vi "Chiller Test Konfig.vi"() -> ()   [LabVIEW 2020, in "EPA 1065.lvlib" / "Chiller NO2 1065-376.lvlib"]
uses:
  Chiller NO2 1065-376.lvlib
  Allgemein/allgemeine Sub-VIs.lvlib
  Seiten/FT-IR/FT-IR.lvlib
  Seiten/FT-IR/FGV FT-IR Gasliste Aktionen.ctl
  Messdaten/Aktionen FGV Messdaten.ctl
  Messdaten/Messdaten.lvlib
  Seiten/Grafik/Grafik.lvlib
  EPA 1065.lvlib
  Allgemeine VIs/Aktion Wertaenderung Gasliste.ctl
  Allgemeine VIs/Aktion Test Status.ctl
  Sprachverwaltung/Sprachverwaltung.lvlib
  Sprachverwaltung/FGV Aktion Tabelle zerlegen.ctl
  Aktion FGV Chiller Test.ctl
  Allgemeine VIs/Aktion Registerkarten ein-ausblenden.ctl
  Funktionstasten/Funktionstasten.lvlib
  Funktionstasten/Funktionstasten-Aktion.ctl
  Funktionstasten/Zustaende.ctl
  T90 1065-308/Ergebnis.ctl
  T90 1065-308/T90 Test 1065-308.lvlib
  PDF_Interface/PDF Interface Helper/PDFResultPictures.ctl
  PDF_Interface/PDF Interface Helper/PDF Interface Helper.lvlib
  Visualisierungs Elemente/Zahlen-Ausgabefeld.ctl
  Visualisierungs Elemente/Auswahlfeld.ctl
  Chiller Konfig Daten.ctl
  Messdaten.ctl
panel:
  out "Ergebnis PDF FALSE":T1 caption="Ergebnis 2"
  out "Ergebnis PDF TRUE":T1 caption="Ergebnis 1"
  out "Daten":T2
  out "Messdaten":sgl[](array[numeric])
  in  "Gasliste geändert":bool
  in  "Registerkarte":T3(tab)
  in  "Abbrechen":bool caption="Cancel"
  in  "Test Start":bool
  in  "Chiller Konfig Daten":T4={"Bearbeiter:"="", "Gasflaschen Nr.:"="", "Accuracy"=0.0, "Sollwert"=0.0, "Messgerät:"="", "Seriennummer:"="", "Pfad:"=path "D:/IAG_Data/Log", "Textname:"="", "Einheit"="", "Expiry Date"=timestamp(0 s since 1904-01-01), "Water Concentration:"=0.0, "Componente:"=""} caption="T90 Konfig Daten" {"Expiry Date" format="%<%x>T"}
  in  "Speichern":bool caption="Save"
  out "NOx":T5=1 caption="Gas 4"
  out "Mwert NOx":sgl caption="Mwert" format="%.3f"
  out "PMwert NOx":sgl caption="PMwert" format="%.3f"
  out "NOx":T6 caption="Konzentration" format="%#.3f"
  out "Graph NOx":waveform(dbl)(graph) caption="Graph1"
  out "NO2":T5=1 caption="Gas 4"
  out "Mwert NO2":sgl caption="Mwert" format="%.3f"
  out "PMwert NO2":sgl caption="PMwert" format="%.3f"
  out "NO2":T6 caption="Konzentration" format="%#.3f"
  out "Graph NO2":waveform(dbl)(graph) caption="Graph1"
  in  "xNOxRef aufzeichnen":bool caption="Test Start"
  out "Countdown Anzeige 2":dbl format="%<%M:%S>T"
  in  "H2O aufgeschalten":bool caption="Test Start"
  out "Timeline":u8(slide) scale=0.0..30.0
  out "Countdown Anzeige":dbl format="%<%M:%S>T"
  out "H2O":T5=1 caption="Gas 4"
  out "Mwert H2O":sgl caption="Mwert" format="%.3f"
  out "PMwert H2O":sgl caption="PMwert" format="%.3f"
  out "H2O 2":T6 caption="Konzentration" format="%#.3f"
  out "Graph H2O":waveform(dbl)(graph) caption="Graph1"
  out "NOx 2":T5=1 caption="Gas 4"
  out "Mwert NOx 2":sgl caption="Mwert" format="%.3f"
  out "PMwert NOx 2":sgl caption="PMwert" format="%.3f"
  out "NOx 2":T6 caption="Konzentration" format="%#.3f"
  out "Graph NOx 2":waveform(dbl)(graph) caption="Graph1"
  out "Mwert H2O 2":sgl caption="Mwert" format="%.3f"
  out "PMwert H2O 2":sgl caption="PMwert" format="%.3f"
  out "H2O 2":T6 caption="Konzentration" format="%#.3f"
  out "Graph H2O 2":waveform(dbl)(graph) caption="Graph1"
  in  "xNOxmeas aufzeichnen":bool caption="Test Start"
  out "Countdown Anzeige 3":dbl format="%<%M:%S>T"
  out "H2O":string caption="%"
  out "xNOxmeas":string caption="ppm"
  out "Ergebnis 1":T1
  out "xNOxmeas_dry":string caption="ppm"
  out "xNOxRef":string caption="ppm"
  out "Ergebnis:":string caption="Result:"
  in  "Print PDF":bool caption="Cancel"
  # "Chiller Test EPA CRF40 §1065.376"
  # "General Settings"
  # "Protocol Settings"
  # "%"
  # "%"
  # "NOx"
  # "±"
  # "x"
  # "NO2"
  # "±"
  # "x"
  # "Saturate the gas cooler with H2O by applying vapor to the measuring input and push the button \"H2O connected\""
  # "H2O"
  # "±"
  # "x"
  # "NOx"
  # "±"
  # "x"
  # "H2O"
  # "±"
  # "x"
  # "xNOxmeas_dry ="
  # "/"
  # "(1-"
  # "/ 100)"
  # "x 0.95"
  # "<"
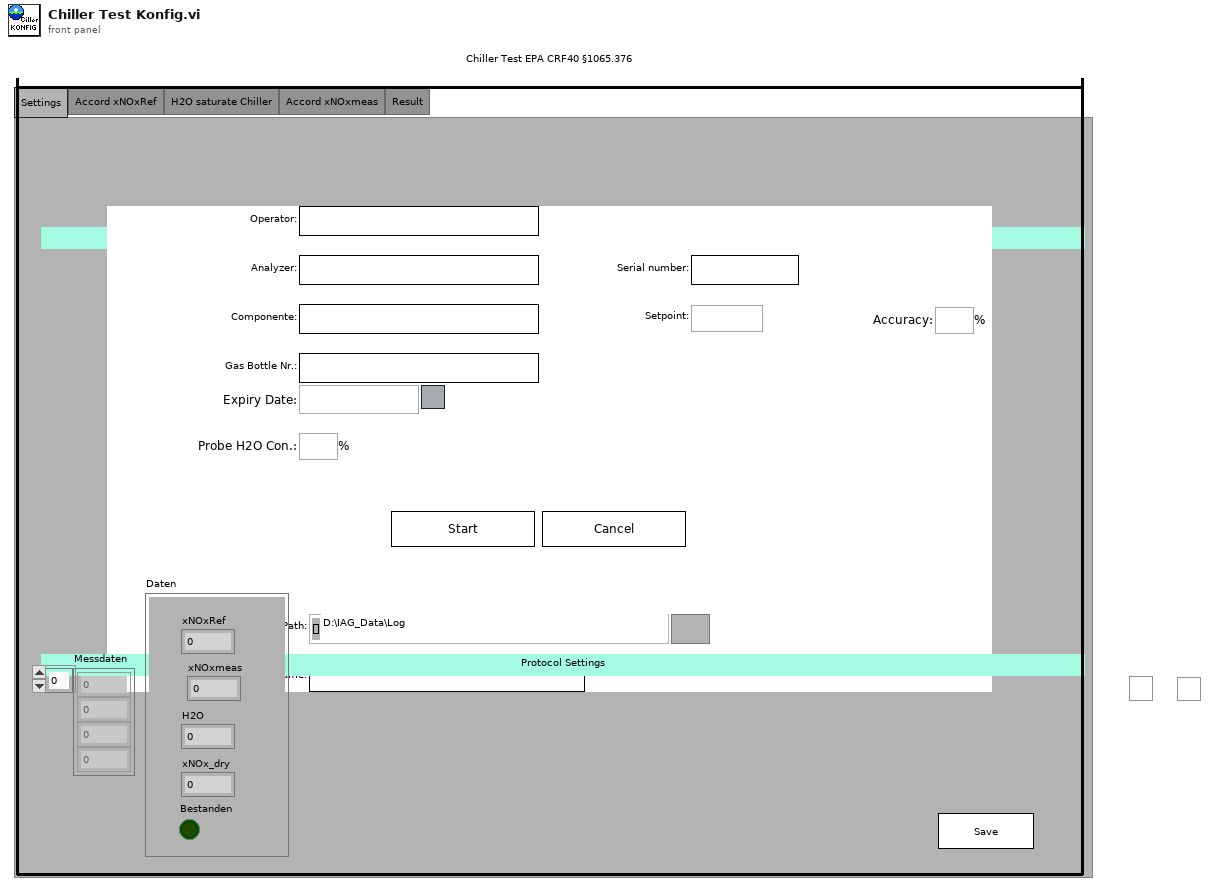
[diagram p1: front panel]
types:
  T1 = typedef "EPA 1065.lvlib/T90 Test 1065-308.lvlib/Ergebnis.ctl" = bool
  T2 = typedef "EPA 1065.lvlib/Chiller NO2 1065-376.lvlib/Messdaten.ctl" = cluster{"xNOxRef":dbl, "xNOxmeas":dbl, "H2O":dbl, "xNOx_dry":dbl, "Bestanden":bool}
  T3 = enum32{"Settings", "Accord xNOxRef", "H2O saturate Chiller", "Accord xNOxmeas", "Result"}
  T4 = typedef "EPA 1065.lvlib/Chiller NO2 1065-376.lvlib/Chiller Konfig Daten.ctl" = cluster{"Bearbeiter:":string, "Gasflaschen Nr.:":string, "Accuracy":dbl, "Sollwert":dbl, "Messgerät:":string, "Seriennummer:":string, "Pfad:":path, "Textname:":string, "Einheit":string, "Expiry Date":timestamp, "Water Concentration:":dbl, "Componente:":string}
  T5 = typedef "Auswahlfeld.ctl" = u16
  T6 = typedef "Zahlen-Ausgabefeld.ctl" = sgl
  T7 = typedef "EPA 1065.lvlib/Chiller NO2 1065-376.lvlib/Aktion FGV Chiller Test.ctl" = enum16{"lesen", "Konfig Daten", "Messdaten", "Resultat", "Daten löschen", "PDF einstellen", "laden", "speichern"}
  T8 = typedef "FT-IR.lvlib/FGV FT-IR Gasliste Aktionen.ctl" = enum16{"lesen", "Gasliste FT-IR", "Gasliste ausgelesen", "laden", "speichern", "löschen"}
  T9 = typedef "EPA 1065.lvlib/Aktion Registerkarten ein-ausblenden.ctl" = enum16{"init", "alle ausblenden", "Seite einblenden", "alle einblenden", "Seite deaktivieren", "Seiten aktivieren"}
  T10 = typedef "Sprachverwaltung.lvlib/FGV Aktion Tabelle zerlegen.ctl" = enum16{"laden", "vereinzeln", "speichern"}
  T11 = typedef "PDF Interface.lvlib/PDF Interface Helper.lvlib/PDFResultPictures.ctl" = cluster{"Yes Ctl Refnum":refnum<vi>, "No Ctl Refnum":refnum<vi>}
  T12 = typedef "String - Ausgabefeld.ctl" = string
  T13 = typedef "EPA 1065.lvlib/Aktion Test Status.ctl" = enum16{"init", "lesen", "prüfen", "Interference 366", "Interference 375", "Chiller läuft", "Drift läuft", "Pre Test läuft", "FID Optimization läuft", "FID Interference läuft", "HovaCAL Interference", "LinV2"}
  T14 = typedef "EPA 1065.lvlib/Aktion Wertaenderung Gasliste.ctl" = enum16{"Init", "lesen", "Gasliste geändert", "ARN inaktiv", "LEAK inaktiv", "Interference 366 inaktiv", "T90 inaktiv", "Interference 375 inaktiv", "Chiller inaktiv", "FID O2 inaktiv", "FID Opti inaktiv", "Drift inaktiv", "Pre Test inaktiv", "LinV2 inaktiv", "HovaCAL Interference inaktiv"}
  T15 = typedef "Messdaten.lvlib/Aktionen FGV Messdaten.ctl" = enum16{"lesen", "schreiben", "löschen", "Mittelwerte", "Komponente"}
  T16 = typedef "Funktionstasten.lvlib/Zustaende.ctl" = enum16{"Standby", "Pause", "Eco", "Messen", "Kalibrieren", "Spülen Filter", "Spülen Leitung", "Umgebungsluft", "0-Gas", "Cal-Gas", "CG zu PNS", "-------------", "Init 1", "Init 2", "Init 3", "Init 4", "Messen vorbereiten", "Messen durchführen", "Exit"}
  T17 = typedef "Funktionstasten.lvlib/Funktionstasten-Aktion.ctl" = enum16{"Initialisieren", "Zustand setzen", "Taste gedrückt", "Fehler speichern", "Lesen", "Manuell", "Remote", "Bitparallel", "Samplepoint", "Zeit Prüfen", "reset Umschalten"}
  T18 = typedef "EPA 1065.lvlib/Aktive Tests Cluster.ctl" = cluster{"ANR läuft":bool, "T90 läuft":bool, "Leak läuft":bool, "Interference 366 läuft":bool, "Interference 375 läuft":bool, "Chiller läuft":bool, "FID Interference läuft":bool, "FID optimization läuft":bool, "Drift läuft":bool, "Pre-test läuft":bool, "HovaCAL Interference läuft":bool, "LinV2 läuft":bool}
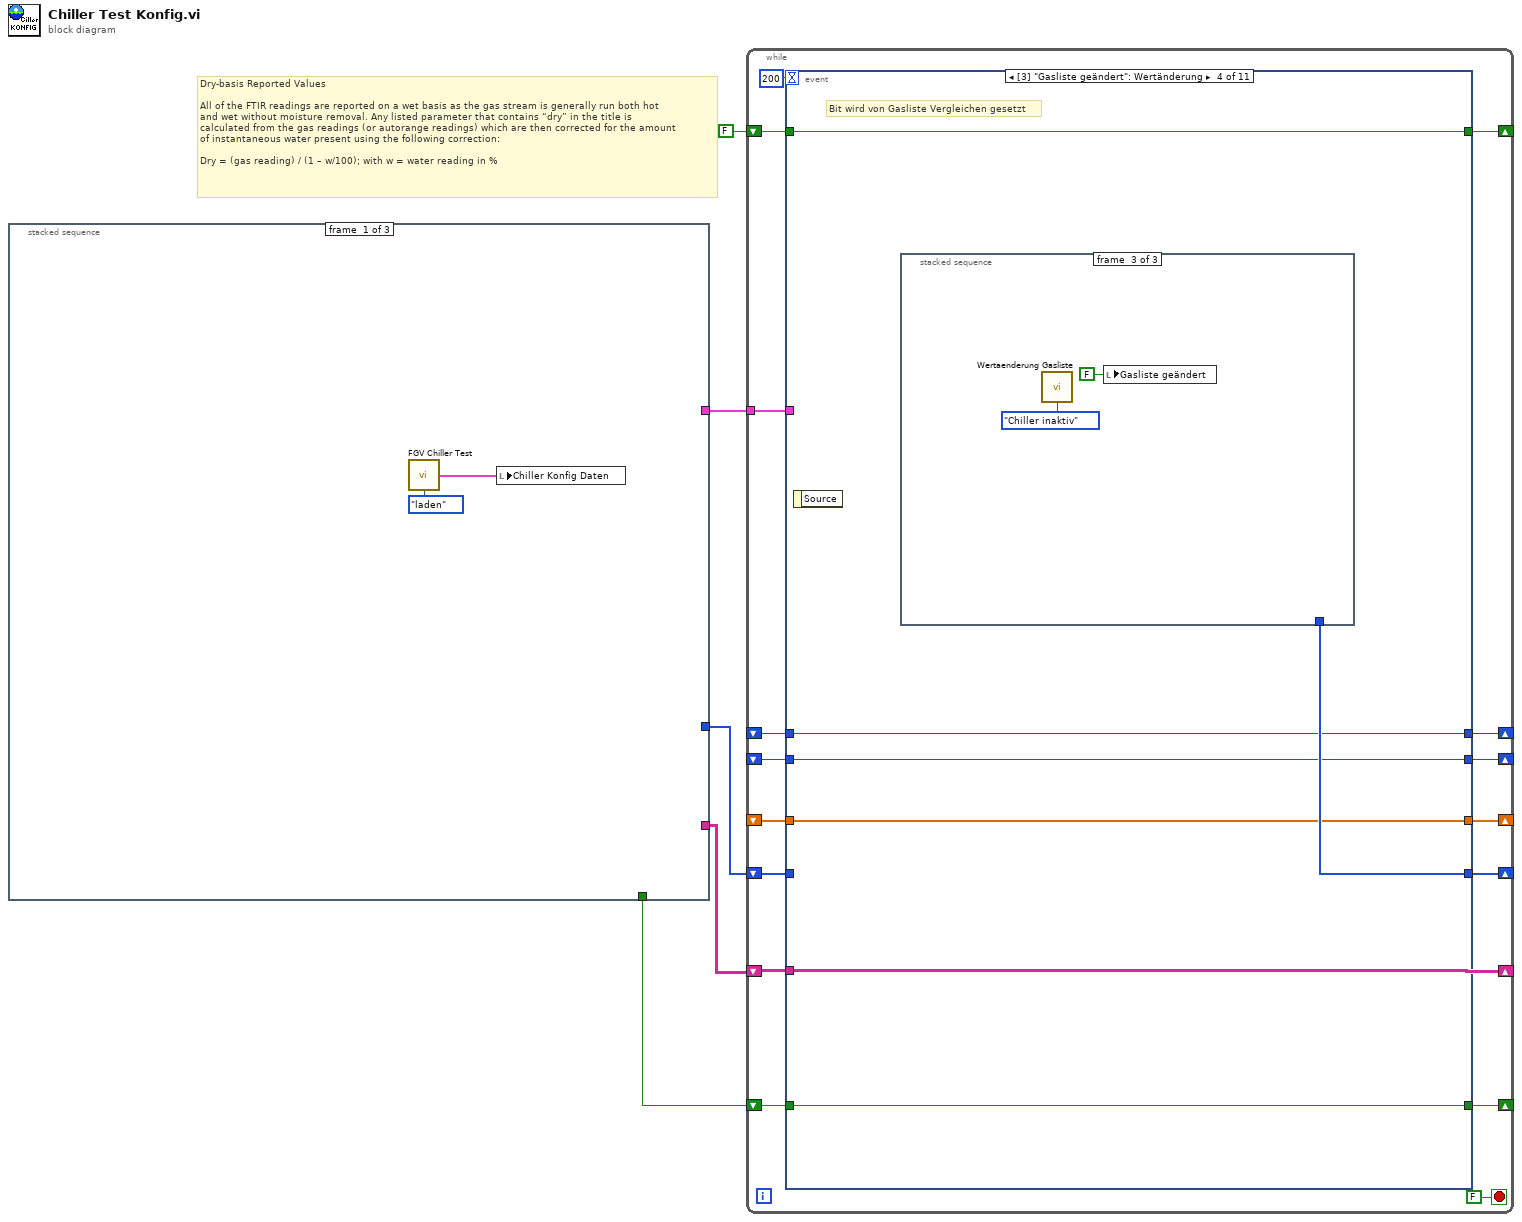
[diagram p0: block diagram]
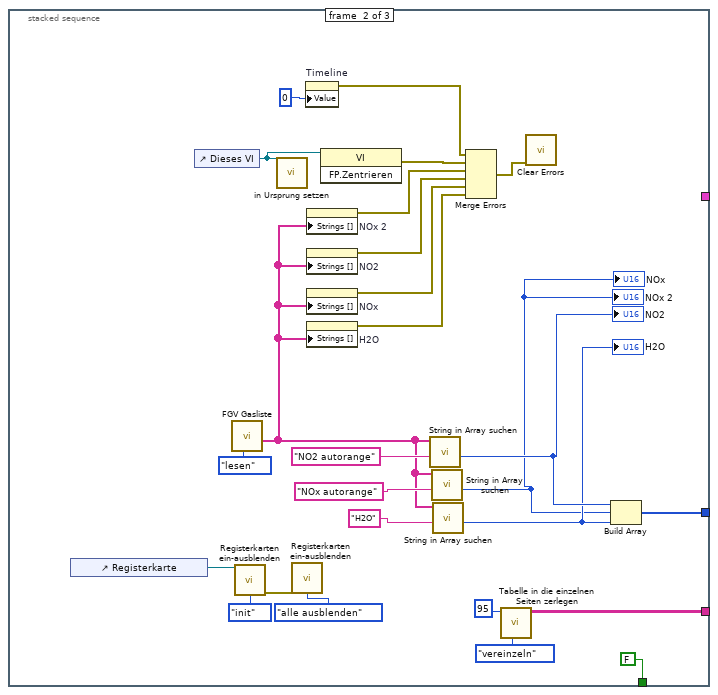
[diagram p2: hidden frame]
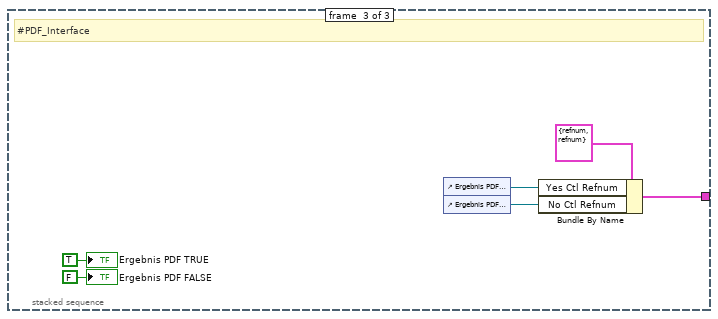
[diagram p3: hidden frame]
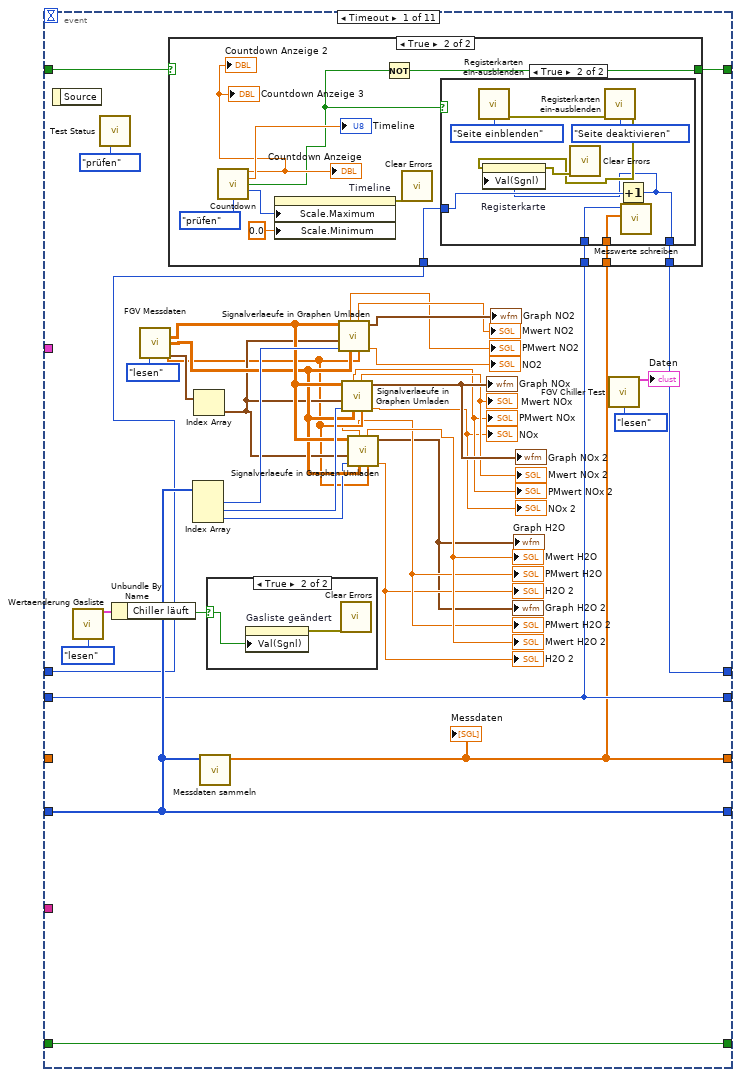
[diagram p4: hidden frame]
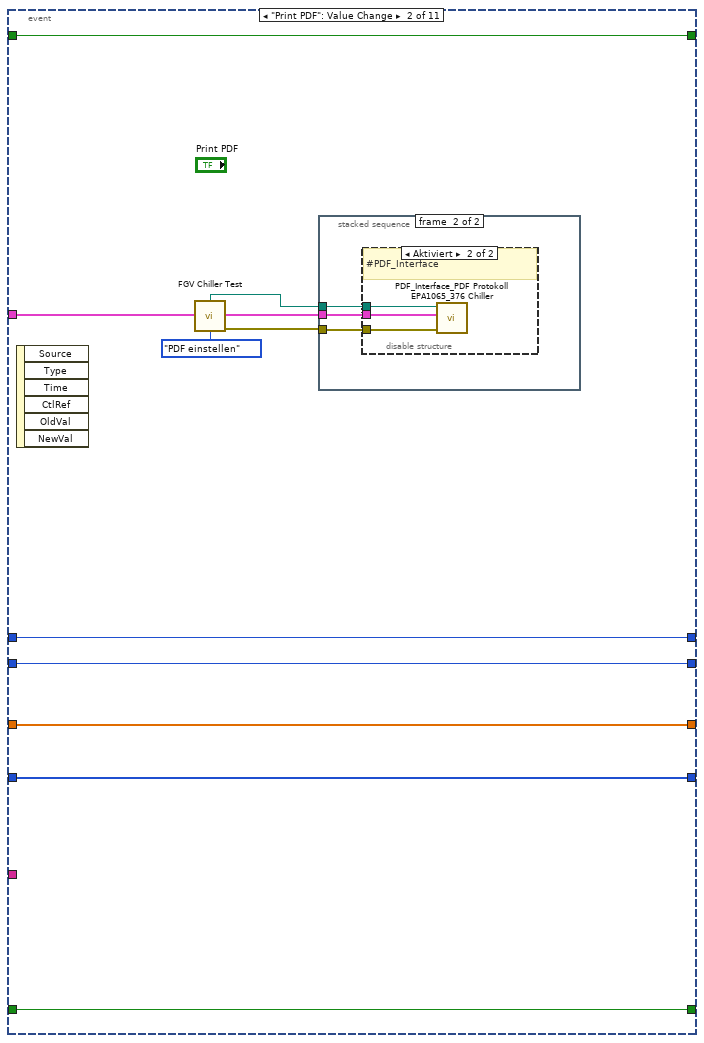
[diagram p8: hidden frame]
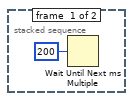
[diagram p9: hidden frame]
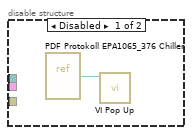
[diagram p10: hidden frame]
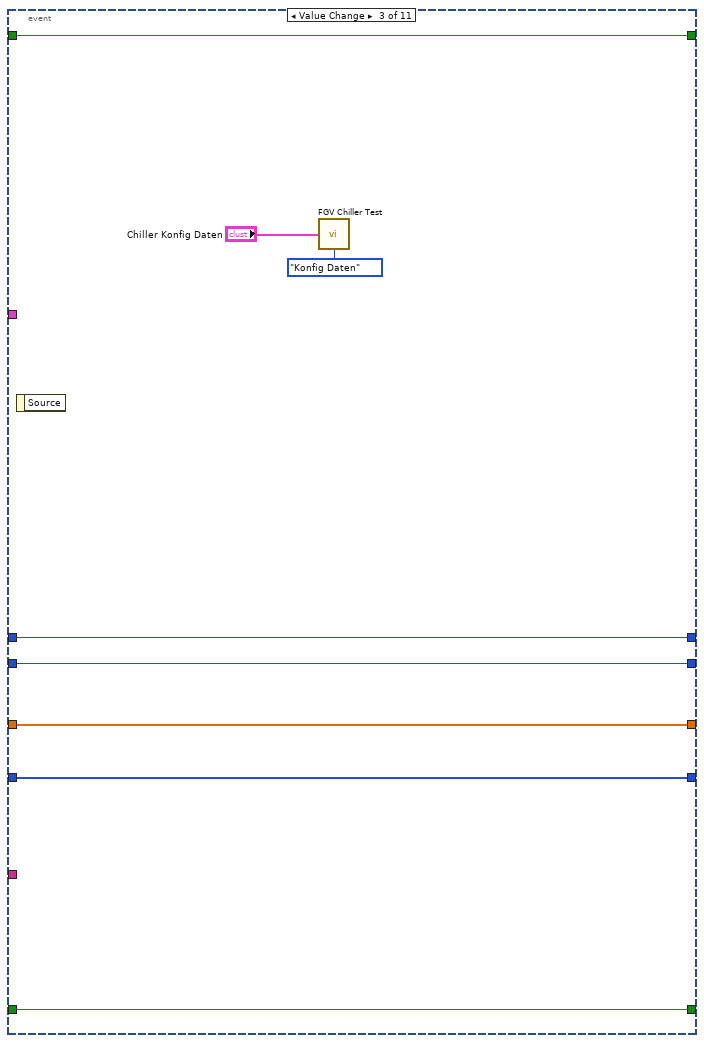
[diagram p11: hidden frame]
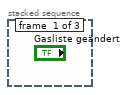
[diagram p12: hidden frame]
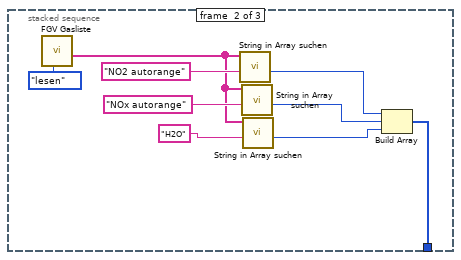
[diagram p13: hidden frame]
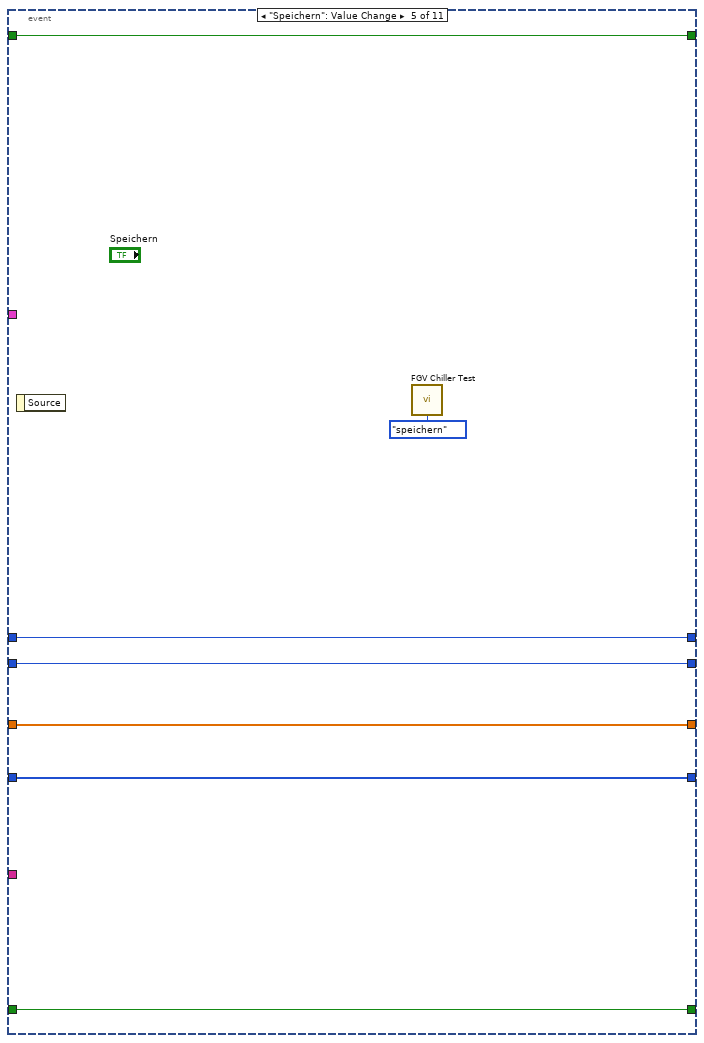
[diagram p14: hidden frame]
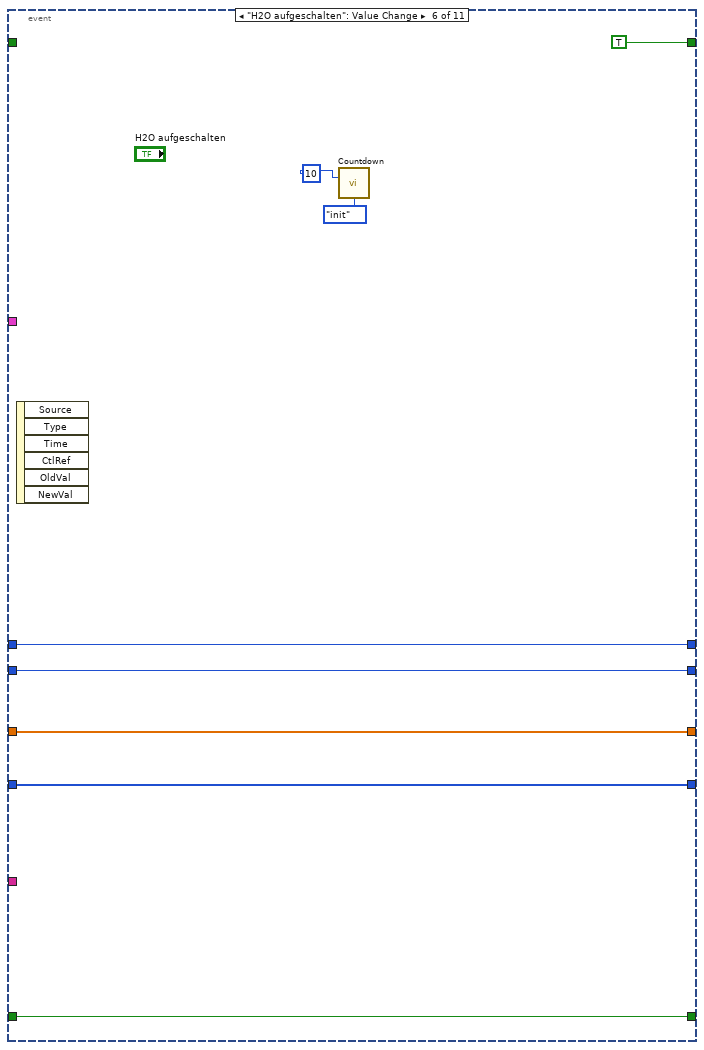
[diagram p15: hidden frame]
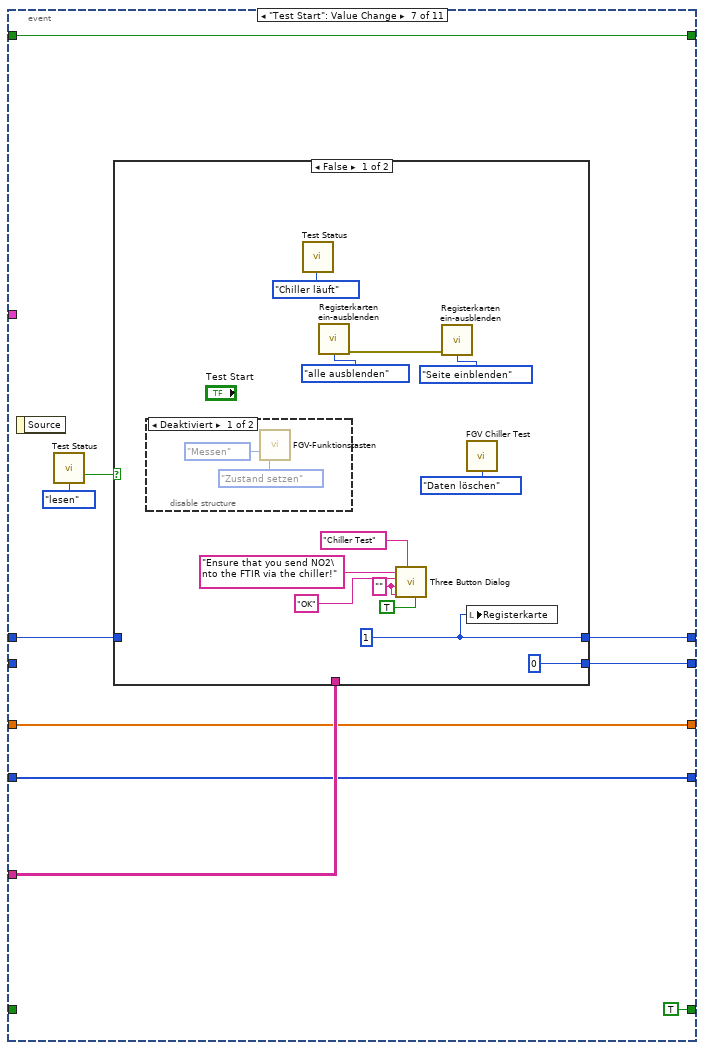
[diagram p16: hidden frame]
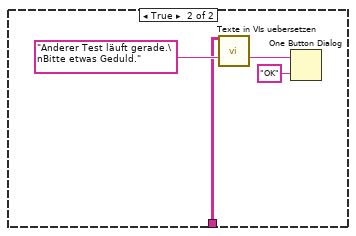
[diagram p18: hidden frame]
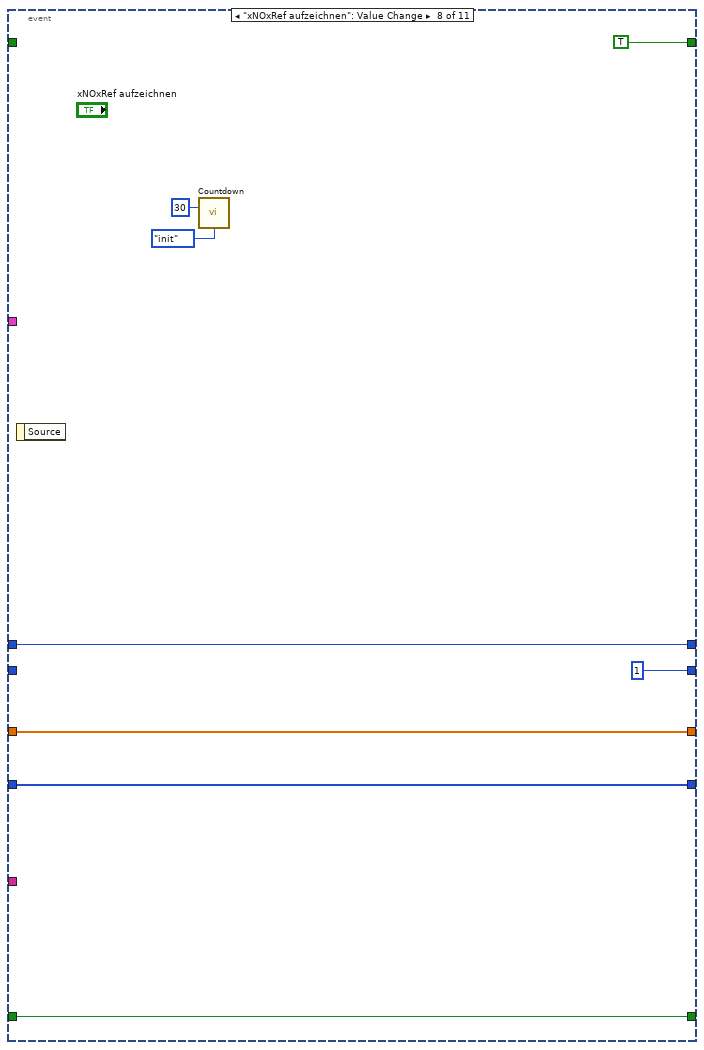
[diagram p19: hidden frame]
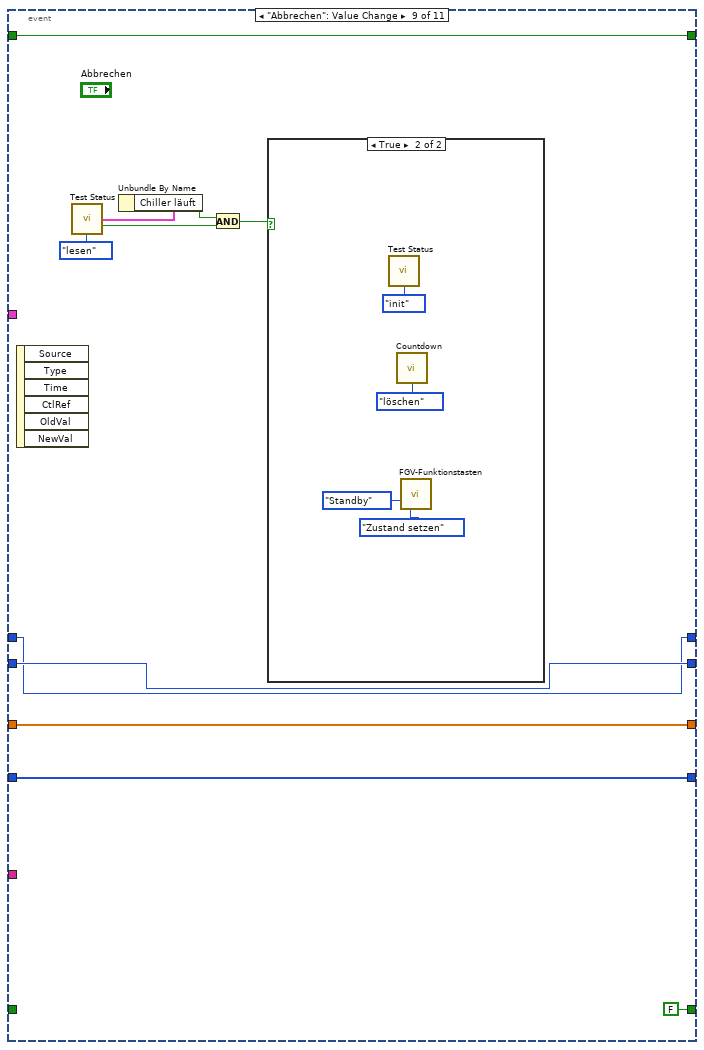
[diagram p20: hidden frame]
diagram:
  # "Dry-basis Reported Values\n\nAll of the FTIR readings are reported on a wet basis as the gas stream is generally run both hot\nand wet without moisture removal. Any listed parameter that contains “dry” in the title is\ncalculated from the gas readings (or autorange readings) which are then corrected for the amount\nof instantaneous water present using the following correction:\n\nDry = (gas reading) / (1 – w/100); with w = water reading in %"
  n1 = stacked-sequence {
    tunnel: [_ w28 _] -> w5
    tunnel: [_ w17 _] -> w3
    tunnel: [_ FALSE _] -> w2
    tunnel: [_ _ w34] -> w1
    frame #0 {
      n2 = call "FGV Chiller Test.vi"("Aktion"=Aktion_FGV_Chiller_Test."laden") -> ("Chiller Konfig Daten"=w6:T4)  [unwired: 11 in, 3 out]
      n3 = local write "Chiller Konfig Daten"(w6) -> ()
    }
    frame #1 {
      n4 = control-ref of="Registerkarte"() -> (w24:refnum<vi>)
      n5 = control-ref of="Dieses VI"() -> (w32:refnum<vi>)
      n6 = call "FGV Gasliste.vi"("Aktionen"=FGV_FT-IR_Gasliste_Aktionen."lesen") -> ("Aktuelle Gasliste gesamt"=w16:T12[])  [unwired: 8 in, 2 out]
      n7 = call "Registerkarten ein-ausblenden.vi"("Registerkartenreferenz"=w24, "Aktion"=Aktion_Registerkarten_ein-ausblenden."init") -> ("error out"=w22:errorcluster)  [unwired: 13 in]
      n8 = call "in Ursprung setzen.vi"("VI Referenz"=w32) -> ()  [unwired: 10 in, 1 out]
      n9 = call "Registerkarten ein-ausblenden.vi"("error in (no error)"=w22, "Aktion"=Aktion_Registerkarten_ein-ausblenden."alle ausblenden") -> ()  [unwired: 13 in, 1 out]
      n10 = property on="Timeline" class="Schieber (strikt)"("Value"=u8 0 ("Timeline")) -> (error out=w26:errorcluster)  [unwired: 2 in, 1 out]
      n11 = property on="NOx 2" class="Ring (strikt)"("Strings []"=w16) -> (error out=w15:errorcluster)  [unwired: 2 in, 1 out]
      n12 = property on="NO2" class="Ring (strikt)"("Strings []"=w16) -> (error out=w14:errorcluster)  [unwired: 2 in, 1 out]
      n13 = property on="NOx" class="Ring (strikt)"("Strings []"=w16) -> (error out=w13:errorcluster)  [unwired: 2 in, 1 out]
      n14 = property on="H2O" class="Ring (strikt)"("Strings []"=w16) -> (error out=w12:errorcluster)  [unwired: 2 in, 1 out]
      n15 = invoke class="VI" method="FP.Zentrieren"(reference=w32) -> (error out=w31:errorcluster)  [unwired: 2 in, 2 out]
      n16 = call "String in Array suchen.vi"("Nach String/Zeichen suchen (-)"="NO2 autorange", "String-Array"=w16) -> ("Index"=w11:i32)  [unwired: 7 in, 2 out]
      "NO2" <- w11
      n17 = call "String in Array suchen.vi"("Nach String/Zeichen suchen (-)"="NOx autorange", "String-Array"=w16) -> ("Index"=w8:i32)  [unwired: 7 in, 2 out]
      "NOx 2" <- w8
      "NOx" <- w8
      n18 = call "String in Array suchen.vi"("Nach String/Zeichen suchen (-)"="H2O", "String-Array"=w16) -> ("Index"=w10:i32)  [unwired: 7 in, 2 out]
      "H2O" <- w10
      n19 = Merge Errors(w26, w31, w15, w14, w13, w12) -> (w33:errorcluster)
      n20 = call "Tabelle in die einzelnen Seiten zerlegen.vi"("Aktion"=FGV_Aktion_Tabelle_zerlegen."vereinzeln", "Index (Seite)"=95) -> ("Sprachliste"=w28:string[][])  [unwired: 7 in, 2 out]
      n21 = call <vilib>:"Clear Errors.vi"("error in (no error)"=w33) -> ()  [unwired: 5 in, 2 out]
      n22 = Build Array(w11, w8, w10) -> (w17:i32[])
    }
    frame #2 {
      # "#PDF_Interface"
      n23 = control-ref of="Ergebnis PDF TRUE"() -> (w36:refnum<vi>)
      n24 = control-ref of="Ergebnis PDF FALSE"() -> (w35:refnum<vi>)
      n25 = Bundle By Name(cluster=T11 {"Yes Ctl Refnum"=refnum, "No Ctl Refnum"=refnum} ("ResultPictures"), "Yes Ctl Refnum"=w36, "No Ctl Refnum"=w35) -> (w34:T11)
      "Ergebnis PDF TRUE" <- T1 TRUE ("Ergebnis PDF TRUE")
      "Ergebnis PDF FALSE" <- T1 FALSE ("Ergebnis PDF FALSE")
    }
  }
  n26 = while {
    shift-right: [w53] -> _
    shift-left: w5 -> [w53]
    shift-right: [w51] -> _
    shift-left: FALSE -> [w52]
    shift-right: [w49] -> _
    shift-left: w3 -> [w50]
    shift-right: [w48] -> _
    shift-left: _ -> [w47]
    shift-right: [w46] -> _
    shift-left: _ -> [w45]
    shift-right: [w44] -> _
    shift-left: _ -> [w43]
    shift-right: [w41] -> _
    shift-left: w2 -> [w42]
    tunnel: w1 -> [w40]
    stop <- FALSE stop-if-true
    n27 = event shown="[3] \"Gasliste geändert\": Wertänderung" {
      selector: _ -> [_ _ _ _ _ _ _ _ _ _ _]
      dyn-events: _ -> [_ _ _ _ _ _ _ _ _ _ _]
      timeout: 200 -> [_ _ _ _ _ _ _ _ _ _ _]
      tunnel: w53 -> [_ _ _ _ _ _ w182 _ _ _ _]
      tunnel: w52 -> [w86 w126 w142 w148 w166 _ w179 _ w216 _ w241]
      tunnel: [w85 w126 w142 w148 w166 TRUE w179 TRUE w216 TRUE w241] -> w51
      tunnel: w50 -> [w84 w125 w139 _ w165 w173 w181 w210 w215 w233 w240]
      tunnel: [w84 w125 w139 w147 w165 w173 w181 w210 w215 w233 w240] -> w49
      tunnel: [w61 w124 w138 w146 w164 w172 w180 w208 w214 w232 w239] -> w48
      tunnel: w47 -> [_ w124 w138 w146 w164 w172 w180 w208 w214 w232 w239]
      tunnel: [w62 w123 w137 w145 w163 w171 w178 1 w213 2 w238] -> w46
      tunnel: w45 -> [w62 w123 w137 w145 w163 w171 _ _ w213 _ w238]
      tunnel: [w60 w120 w136 w144 w161 w168 w177 w204 w212 w227 w234] -> w44
      tunnel: w43 -> [w57 w120 w136 w144 w161 w168 w175 w204 w212 w227 w234]
      tunnel: w42 -> [w56 w119 w135 w143 w160 w167 _ w203 _ w226 w237]
      tunnel: [w56 w119 w135 w143 w160 w167 TRUE w203 FALSE w226 w236] -> w41
      tunnel: w40 -> [_ w117 _ _ _ _ _ _ _ _ _]
      event Timeout {
        n28 = event-data() -> ()  [unwired: 1 in, 1 out]
        n29 = call "Wertaenderung Gasliste.vi"("Aktion"=Aktion_Wertaenderung_Gasliste."lesen") -> ("Tests"=w87:T18)  [unwired: 13 in, 1 out]
        n30 = call "Test Status.vi"("Aktion"=Aktion_Test_Status."prüfen") -> ()  [unwired: 11 in, 4 out]
        n31 = Unbundle By Name(w87) -> ("Chiller läuft"=w63:bool)
        n32 = call "FGV Messdaten.vi"("Aktionen"=Aktionen_FGV_Messdaten."lesen") -> ("Messdaten"=w81:sgl[][], "Mittelwertdaten"=w80:sgl[][], "Deviation"=w77:sgl[], "Zeitstempeln"=w90:timestamp[])  [unwired: 6 in, 5 out]
        n33 = Index Array(array=w84) -> (element #1=w83:i32, element #2=w82:i32, element #3=w78:i32)  [unwired: 3 in]
        n34 = Index Array(array=w90) -> (element=w79:timestamp)  [unwired: 1 in]
        n35 = call "Messdaten sammeln.vi"("Gasindex"=w84) -> ("Messdaten"=w61:sgl[])  [unwired: 9 in, 1 out]
        "Messdaten" <- w61
        n36 = case shown="True" w86 {
          selector: w86 -> [w92 _]
          tunnel: [w92 w100] -> w85
          tunnel: w62 -> [_ w97]
          tunnel: w61 -> [_ w96]
          tunnel: [w91 w95] -> w60
          tunnel: w57 -> [w91 w94]
          frame False {
          }
          frame True {
            n37 = call "Countdown.vi"("Aktion"=enum16{"init", "prüfen", "löschen"}."prüfen") -> ("Countdown Anzeige"=→"Countdown Anzeige" →"Countdown Anzeige 2" →"Countdown Anzeige 3":dbl, "Laufleiste"=→"Timeline":dbl, "Zeit abgelaufen"=w93:bool, "Laufleistenbereich"=w104:u32)  [unwired: 10 in, 1 out]
            n38 = property on="Timeline" class="Schieber (strikt)"("Scale.Maximum"=w104, "Scale.Minimum"=0.0 ("Skala.Bereich:Minimum")) -> (error out=w101:errorcluster)  [unwired: 2 in, 1 out]
            n39 = Not(x=w93) -> (.not. x?=w100:bool)
            n40 = call <vilib>:"Clear Errors.vi"("error in (no error)"=w101) -> ()  [unwired: 5 in, 2 out]
            n41 = case shown="True" w93 {
              tunnel: w97 -> [_ w111]
              tunnel: w96 -> [_ w110]
              tunnel: [w105 w106] -> w95
              tunnel: w94 -> [w105 w109]
              frame False {
              }
              frame True {
                n42 = call "Registerkarten ein-ausblenden.vi"("Aktion"=Aktion_Registerkarten_ein-ausblenden."Seite einblenden") -> ("error out"=w112:errorcluster)  [unwired: 14 in]
                n43 = call "Registerkarten ein-ausblenden.vi"("error in (no error)"=w112, "Aktion"=Aktion_Registerkarten_ein-ausblenden."Seite deaktivieren") -> ("error out"=w107:errorcluster)  [unwired: 13 in]
                n44 = Increment(x=w109) -> (x+1=w106:i32)
                n45 = property on="Registerkarte" class="RKElem (strikt)"(error in=w107, "Val(Sgnl)"=w106) -> (error out=w108:errorcluster)  [unwired: 1 in, 1 out]
                n46 = call <vilib>:"Clear Errors.vi"("error in (no error)"=w108) -> ()  [unwired: 5 in, 2 out]
                n47 = call "Messwerte schreiben.vi"("Messdaten"=w110, "Numerisch (Eingang)"=w111) -> ()  [unwired: 9 in, 1 out]
              }
            }
          }
        }
        n48 = case shown="True" w63 {
          selector: w63 -> [_ w115]
          frame False {
          }
          frame True {
            n49 = property on="Gasliste geändert" class="Bool. (strikt)"("Val(Sgnl)"=w115) -> (error out=w116:errorcluster)  [unwired: 2 in, 1 out]
            n50 = call <vilib>:"Clear Errors.vi"("error in (no error)"=w116) -> ()  [unwired: 5 in, 2 out]
          }
        }
        n51 = call "Signalverlaeufe in Graphen Umladen.vi"("Deviation"=w77, "Mittelwertdaten"=w80, "Gas-Auswahl"=w83, "t0"=w79, "Werte"=w81) -> ("Konzentration"=→"NO2":sgl, "Waveform"=→"Graph NO2":waveform(dbl), "aktuelle Mittelwert"=→"Mwert NO2":sgl, "Deviation"=→"PMwert NO2":sgl)  [unwired: 2 in, 1 out]
        n52 = call "Signalverlaeufe in Graphen Umladen.vi"("Deviation"=w77, "Mittelwertdaten"=w80, "Gas-Auswahl"=w82, "t0"=w79, "Werte"=w81) -> ("Konzentration"=→"NOx" →"NOx 2":sgl, "Waveform"=→"Graph NOx" →"Graph NOx 2":waveform(dbl), "aktuelle Mittelwert"=→"Mwert NOx" →"Mwert NOx 2":sgl, "Deviation"=→"PMwert NOx" →"PMwert NOx 2":sgl)  [unwired: 2 in, 1 out]
        n53 = call "Signalverlaeufe in Graphen Umladen.vi"("Deviation"=w77, "Mittelwertdaten"=w80, "Gas-Auswahl"=w78, "t0"=w79, "Werte"=w81) -> ("Konzentration"=→"H2O 2" →"H2O 2":sgl, "Waveform"=→"Graph H2O 2" →"Graph H2O":waveform(dbl), "aktuelle Mittelwert"=→"Mwert H2O 2" →"Mwert H2O":sgl, "Deviation"=→"PMwert H2O 2" →"PMwert H2O":sgl)  [unwired: 2 in, 1 out]
        n54 = call "FGV Chiller Test.vi"("Aktion"=Aktion_FGV_Chiller_Test."lesen") -> ("Daten"=→"Daten":T2)  [unwired: 11 in, 3 out]
      }
      event "Print PDF": Value Change {
        n55 = event-data() -> ()  [unwired: 1 in, 6 out]
        n56 = call "FGV Chiller Test.vi"("Aktion"=Aktion_FGV_Chiller_Test."PDF einstellen") -> ("PDF Pfad"=w118:path, "error out"=w121:errorcluster)  [unwired: 11 in, 2 out]
        n57 = stacked-sequence {
          tunnel: w121 -> [_ w130]
          tunnel: w118 -> [_ w129]
          tunnel: w117 -> [_ w128]
          frame #0 {
            n58 = Wait Until Next ms Multiple(millisecond multiple=u32 200 ("ms")) -> ()  [unwired: 1 out]
          }
          frame #1 {
            n59 = disable-structure shown="Aktiviert" {
              disable-tunnel: w130 -> [_ w134]
              disable-tunnel: w129 -> [_ w133]
              disable-tunnel: w128 -> [_ w132]
              frame Disabled {
                n60 = vi-ref "PDF Protokoll EPA1065_376 Chiller.vi"() -> (w131:refnum<vi>)
                n61 = call "VI Pop Up.vi"("VI Referenz"=w131) -> ()  [unwired: 10 in, 1 out]
              }
              frame Enabled {
                # "#PDF_Interface"
                n62 = call "PDF_Interface_PDF Protokoll EPA1065_376 Chiller.vi"("error in (no error)"=w134, "ResultPictures"=w132, "Save PDF File Path"=w133) -> ()  [unwired: 8 in, 1 out]
              }
            }
          }
        }
      }
      event Value Change {
        n63 = event-data() -> ()  [unwired: 1 in, 1 out]
        n64 = call "FGV Chiller Test.vi"("Chiller Konfig Daten"="Chiller Konfig Daten", "Aktion"=Aktion_FGV_Chiller_Test."Konfig Daten") -> ()  [unwired: 10 in, 4 out]
      }
      event "Gasliste geändert": Value Change {
        # "Bit wird von Gasliste Vergleichen gesetzt"
        n65 = event-data() -> ()  [unwired: 1 in, 1 out]
        n66 = stacked-sequence {
          tunnel: [_ w149 _] -> w147
          frame #0 {
          }
          frame #1 {
            n67 = call "FGV Gasliste.vi"("Aktionen"=FGV_FT-IR_Gasliste_Aktionen."lesen") -> ("Aktuelle Gasliste gesamt"=w154:T12[])  [unwired: 8 in, 2 out]
            n68 = call "String in Array suchen.vi"("Nach String/Zeichen suchen (-)"="NO2 autorange", "String-Array"=w154) -> ("Index"=w152:i32)  [unwired: 7 in, 2 out]
            n69 = call "String in Array suchen.vi"("Nach String/Zeichen suchen (-)"="NOx autorange", "String-Array"=w154) -> ("Index"=w151:i32)  [unwired: 7 in, 2 out]
            n70 = call "String in Array suchen.vi"("Nach String/Zeichen suchen (-)"="H2O", "String-Array"=w154) -> ("Index"=w150:i32)  [unwired: 7 in, 2 out]
            n71 = Build Array(w152, w151, w150) -> (w149:i32[])
          }
          frame #2 {
            n72 = call "Wertaenderung Gasliste.vi"("Aktion"=Aktion_Wertaenderung_Gasliste."Chiller inaktiv") -> ()  [unwired: 13 in, 2 out]
            n73 = local write "Gasliste geändert"(FALSE ("Gasliste geändert")) -> ()
          }
        }
      }
      event "Speichern": Value Change {
        n74 = event-data() -> ()  [unwired: 1 in, 1 out]
        n75 = call "FGV Chiller Test.vi"("Aktion"=Aktion_FGV_Chiller_Test."speichern") -> ()  [unwired: 11 in, 4 out]
      }
      event "H2O aufgeschalten": Value Change {
        n76 = event-data() -> ()  [unwired: 1 in, 6 out]
        n77 = call "Countdown.vi"("sec"=u32 10 ("Min"), "Aktion"=enum16{"init", "prüfen", "löschen"}."init") -> ()  [unwired: 9 in, 5 out]
      }
      event "Test Start": Value Change {
        n78 = event-data() -> ()  [unwired: 1 in, 1 out]
        n79 = call "Test Status.vi"("Aktion"=Aktion_Test_Status."lesen") -> ("Tests sperren"=w183:bool)  [unwired: 11 in, 3 out]
        n80 = case shown="False" w183 {
          tunnel: w182 -> [_ w199]
          tunnel: [0 _] -> w178
          tunnel: [w190 _] -> w177
          tunnel: w175 -> [_ _]
          frame False {
            w187 = "" ("Center Button Text (\"No\")")
            w190 = 1
            n81 = disable-structure shown="Deaktiviert" {
              frame Disabled {
                n82 = call "FGV-Funktionstasten.vi"("Zustand"=Zustaende."Messen", "Aktion"=Funktionstasten-Aktion."Zustand setzen") -> ()  [unwired: 6 in, 8 out]
              }
              frame Enabled {
              }
            }
            n83 = call "Test Status.vi"("Aktion"=Aktion_Test_Status."Chiller läuft") -> ()  [unwired: 11 in, 4 out]
            n84 = call "Registerkarten ein-ausblenden.vi"("Aktion"=Aktion_Registerkarten_ein-ausblenden."alle ausblenden") -> ("error out"=w194:errorcluster)  [unwired: 14 in]
            n85 = call <vilib>:"Three Button Dialog.vi"("Allow user to close window? (TRUE)"=TRUE, "Window Title (\"\")"="Chiller Test" ("Window Title (\"\")"), "Right Button Text (\"Cancel\")"=w187, "Center Button Text (\"No\")"=w187, "Left Button Text (\"Yes\")"="OK" ("Left Button Text (\"Yes\")"), "message"="Ensure that you send NO2\nto the FTIR via the chiller!" ("Nachricht")) -> ()  [unwired: 5 in, 1 out]
            n86 = call "Registerkarten ein-ausblenden.vi"("error in (no error)"=w194, "Aktion"=Aktion_Registerkarten_ein-ausblenden."Seite einblenden") -> ()  [unwired: 13 in, 1 out]
            n87 = call "FGV Chiller Test.vi"("Aktion"=Aktion_FGV_Chiller_Test."Daten löschen") -> ()  [unwired: 11 in, 4 out]
            n88 = local write "Registerkarte"(w190) -> ()
          }
          frame True {
            n89 = call "Texte in VIs uebersetzen.vi"("Sprachliste"=w199, "String zum Übersetzen"="Anderer Test läuft gerade.\nBitte etwas Geduld." ("Nachricht")) -> ("String zum Übersetzen"=w200:string)  [unwired: 9 in, 4 out]
            n90 = One Button Dialog(message=w200, button name ("OK")="OK" ("Schaltflächentext (\"OK\")")) -> ()  [unwired: 1 out]
          }
        }
      }
      event "xNOxRef aufzeichnen": Value Change {
        n91 = event-data() -> ()  [unwired: 1 in, 1 out]
        n92 = call "Countdown.vi"("sec"=u32 30, "Aktion"=enum16{"init", "prüfen", "löschen"}."init") -> ()  [unwired: 9 in, 5 out]
      }
      event "Abbrechen": Value Change {
        n93 = event-data() -> ()  [unwired: 1 in, 6 out]
        n94 = call "Test Status.vi"("Aktion"=Aktion_Test_Status."lesen") -> ("Aktive Tests"=w220:T18, "Tests sperren"=w218:bool)  [unwired: 11 in, 2 out]
        n95 = Unbundle By Name(w220) -> ("Chiller läuft"=w219:bool)
        n96 = And(x=w219, y=w218) -> (x .and. y?=w217:bool)
        n97 = case shown="True" w217 {
          frame False {
          }
          frame True {
            n98 = call "Test Status.vi"("Aktion"=Aktion_Test_Status."init") -> ()  [unwired: 11 in, 4 out]
            n99 = call "Countdown.vi"("Aktion"=enum16{"init", "prüfen", "löschen"}."löschen") -> ()  [unwired: 10 in, 5 out]
            n100 = call "FGV-Funktionstasten.vi"("Zustand"=Zustaende."Standby", "Aktion"=Funktionstasten-Aktion."Zustand setzen") -> ()  [unwired: 6 in, 8 out]
          }
        }
      }
      event "xNOxmeas aufzeichnen": Value Change {
        n101 = event-data() -> ()  [unwired: 1 in, 1 out]
        n102 = call "Countdown.vi"("sec"=u32 30, "Aktion"=enum16{"init", "prüfen", "löschen"}."init") -> ()  [unwired: 9 in, 5 out]
      }
      event "Registerkarte": Value Change {
        n103 = event-data() -> ()  [unwired: 1 in, 1 out]
        n104 = case shown="\"Settings\", Standard" "Registerkarte" {
          tunnel: w237 -> [w242 w243 w244 w245 w247]
          tunnel: [w242 w243 w244 w245 w246] -> w236
          frame "Settings", Default {
          }
          frame "Accord xNOxRef" {
          }
          frame "H2O saturate Chiller" {
          }
          frame "Accord xNOxmeas" {
          }
          frame "Result" {
            n105 = case shown="True" w247 {
              selector: w247 -> [w248 _]
              tunnel: [w248 FALSE] -> w246
              frame False {
              }
              frame True {
                n106 = call "FGV Chiller Test.vi"("Aktion"=Aktion_FGV_Chiller_Test."Resultat") -> ("Daten"=w262:T2, "error out"=w267:errorcluster)  [unwired: 11 in, 2 out]
                n107 = Unbundle By Name(w262) -> ("xNOxRef"=w261:dbl, "xNOxmeas"=w260:dbl, "H2O"=w259:dbl, "xNOx_dry"=w258:dbl, "Bestanden"=w250:bool)
                "Ergebnis 1" <- w250
                n108 = call "Test Status.vi"("error in (no error)"=w267, "Aktion"=Aktion_Test_Status."init") -> ()  [unwired: 10 in, 4 out]
                n109 = Number To Fractional String(number=w261, precision (6)=i16 2 ("Genauigkeit (6)")) -> (F-format string=→"xNOxRef":string)  [unwired: 2 in]
                n110 = Number To Fractional String(number=w260, precision (6)=i16 2 ("Genauigkeit (6)")) -> (F-format string=→"xNOxmeas":string)  [unwired: 2 in]
                n111 = Number To Fractional String(number=w259, precision (6)=i16 2 ("Genauigkeit (6)")) -> (F-format string=→"H2O":string)  [unwired: 2 in]
                n112 = Number To Fractional String(number=w258, precision (6)=i16 3 ("Genauigkeit (6)")) -> (F-format string=→"xNOxmeas_dry":string)  [unwired: 2 in]
                n113 = Select(t="passed", s=w250, f="failed") -> (s? t:f=→"Ergebnis:":string)
              }
            }
          }
        }
      }
    }
  }
